vi "Grava_PixelReg_u.vi"(2 "Pixel Register programmed":u32[](array[numeric]) format="%x", 3 "Folder path":path) -> (1 "quants arxius fets":i32)   [LabVIEW 2015, in "VIPM2.lvlib"]
doc: "Grava els Pixel Registers programats en arxius personalitzats per ChipID\n\" \\ChipID_PixelReg.txt \""
uses:
  VIPM2.lvlib
panel:
  # "Subrutina: grava els Pixel Registers programats en arxius personalitzats per ChipID"
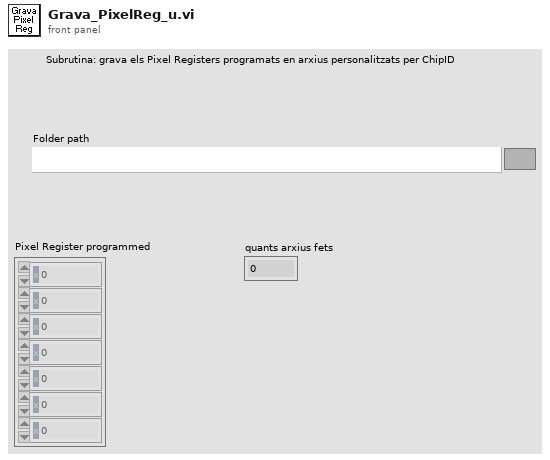
[diagram p1: front panel]
types:
  T1 = enum16{"open", "replace", "create", "open or create", "replace or create", "replace or create with confirmation"}
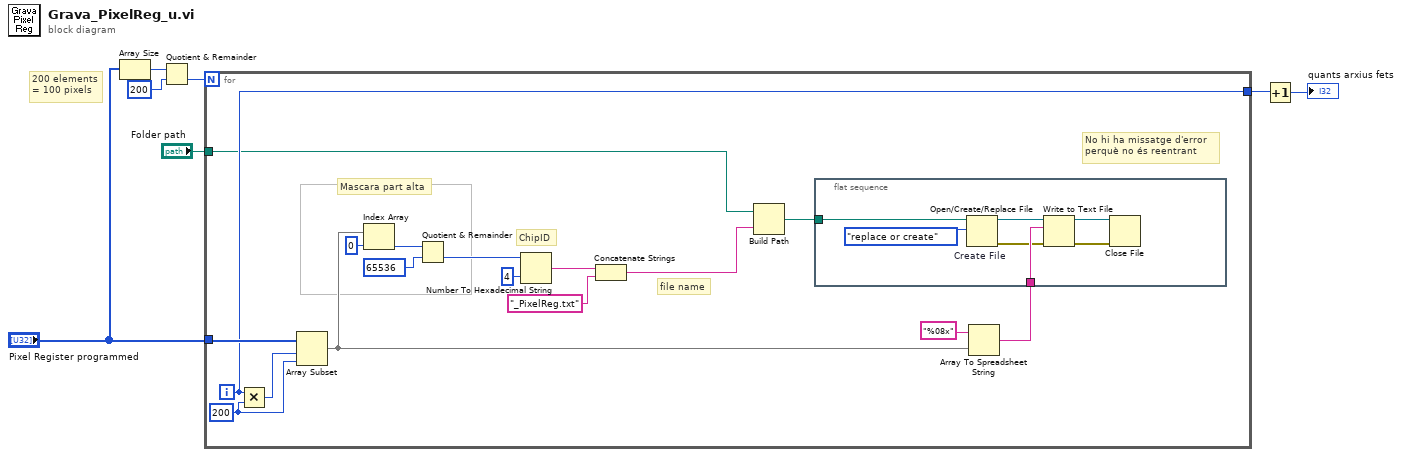
[diagram p0: block diagram]
diagram:
  # "200 elements\n= 100 pixels"
  n1 = Array Size(array="Pixel Register programmed") -> (size(s)=w6:i32)
  n2 = Quotient & Remainder(x=w6, y=200) -> (floor(x/y)=w7:i32)  [unwired: 1 out]
  n3 = for {
    N: w7 -> [_]
    tunnel: "Pixel Register programmed" -> [w24]
    tunnel: [w14] -> w3
    tunnel: "Folder path" -> [w12]
    i -> [w14]
    w22 = 200 ("y")
    # "No hi ha missatge d'error\nperquè no és reentrant"
    # "file name"
    # "ChipID"
    # "Mascara part alta"
    n4 = Multiply(x=w14, y=w22) -> (x*y=w23:i32)
    n5 = Array Subset "Array Subset"(array=w24, index=w23, length=w22) -> (w9:u32[])
    n6 = Index Array "Index Array"(array=w9, index=0) -> (element=w20:u32)
    n7 = Quotient & Remainder(x=w20, y=u32 65536) -> (floor(x/y)=w18:u32)  [unwired: 1 out]
    n8 = Number To Hexadecimal String(1:i16 4 ("width (-)"), 2:w18) -> (0:w16:string)
    n9 = Concatenate Strings "Concatenate Strings"(w16, "_PixelReg.txt" ("string")) -> (w13:string)
    n10 = Build Path(base path=w12, name or relative path=w13) -> (appended path=w8:path)
    n11 = flat-sequence {
      tunnel: w11 -> [w31]
      tunnel: w8 -> [w25]
      frame #0 {
        n12 = Open/Create/Replace File "Create File"(file path (use dialog)=w25, operation (0:open)=T1."replace or create") -> (refnum out=w29:refnum<file>, error out=w28:errorcluster)  [unwired: 4 in, 1 out]
        n13 = Write to Text File(file (use dialog)=w29, text=w31, error in=w28) -> (refnum out=w27:refnum<file>, error out=w26:errorcluster)  [unwired: 1 in, 1 out]
        n14 = Close File(refnum=w27, error in=w26) -> ()  [unwired: 2 out]
      }
    }
    n15 = Array To Spreadsheet String(array=w9, 3:"%08x" ("format (%08x)")) -> (spreadsheet string=w11:string)  [unwired: 1 in]
  }
  n16 = Increment(x=w3) -> (x+1=→"quants arxius fets":i32)
